vi "DGHD5331_timestamp.vi"() -> ()   [LabVIEW 2014]
uses:
  <vilib>/Instr/_visa.llb/VISA Configure Serial Port (Instr).vi
  <vilib>/Utility/file.llb/Write To Spreadsheet File (string).vi
  <vilib>/Utility/file.llb/Write To Spreadsheet File (DBL).vi
panel:
  out "Time/Date":string
  out "Waveform Chart":dynamicdata(graph)
  out "Data Read":string
  out "Exp time (sec)":dbl
  out "Bytes Read":u32
  in  "Comm Port":refnum<visa-resource-name>
  in  "Loop Timer":u32=500 min=500 max=5000 step=500
  in  "stop":bool
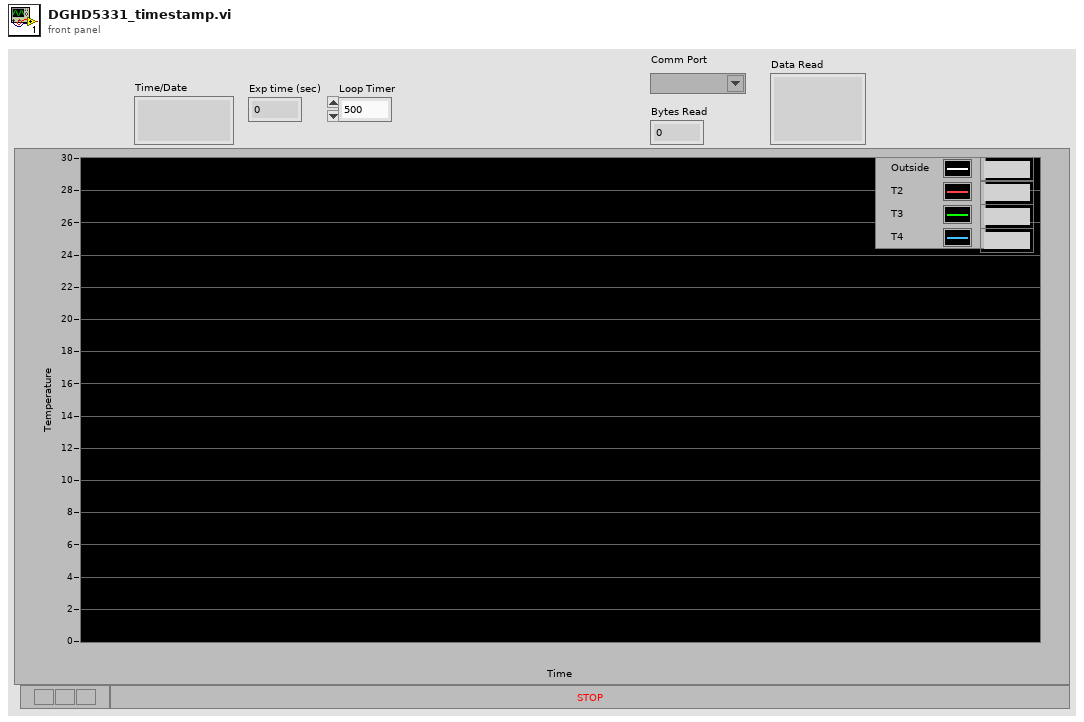
[diagram p1: front panel]
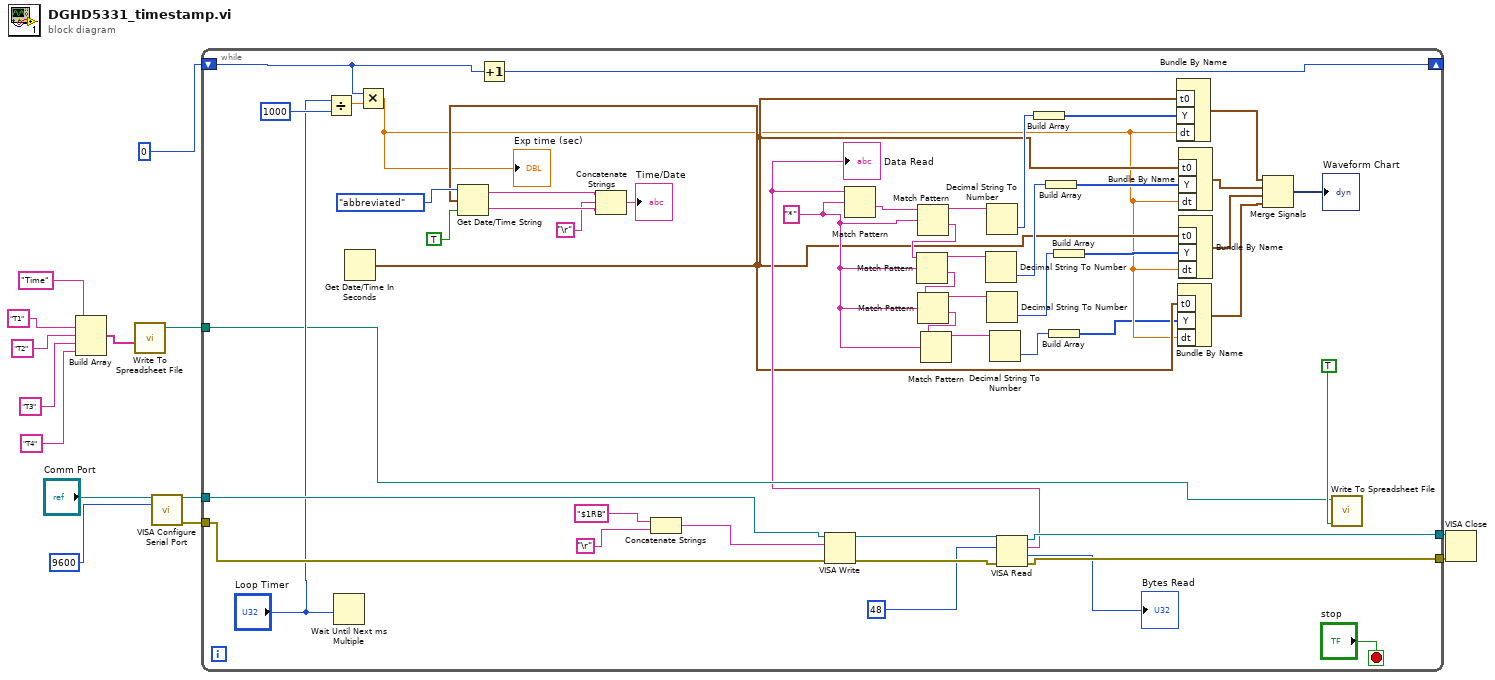
[diagram p0: block diagram]
diagram:
  n1 = Build Array("Time", "T1", "T2", "T3", "T4") -> (w3:string[])
  n2 = call-poly <vilib>:"Write To Spreadsheet File.vi"("1D data"=w3) -> ("new file path (Not A Path if cancelled)"=w1:path)  [unwired: 7 in]
  n3 = call-poly "VISA Configure Serial Port"("VISA resource name"="Comm Port", "baud rate (9600)"=9600) -> ("VISA resource name out"=w13:refnum<visa-resource-name>, "error out"=w11:errorcluster)  [unwired: 12 in]
  n4 = while {
    tunnel: w13 -> [w63]
    tunnel: w11 -> [w62]
    tunnel: [w59] -> w10
    tunnel: [w58] -> w9
    shift-right: [w39] -> _
    shift-left: 0 -> [w50]
    tunnel: w1 -> [w38]
    stop <- "stop" stop-if-true
    w43 = "*"
    n5 = Divide(x="Loop Timer", y=1000) -> (x/y=w52:dbl)
    n6 = Wait Until Next ms Multiple(millisecond multiple="Loop Timer") -> ()  [unwired: 1 out]
    n7 = Get Date/Time In Seconds() -> (seconds since 1Jan1904=w27:timestamp)
    n8 = Multiply(x=w50, y=w52) -> (x*y=w26:dbl)
    "Exp time (sec)" <- w26
    n9 = Get Date/Time String(date format (0)=enum16{"short", "long", "abbreviated"}."abbreviated", seconds (now)=w27, want seconds? (F)=TRUE) -> (date string=w18:string, time string=w17:string)
    n10 = Increment(x=w50) -> (x+1=w39:i32)
    n11 = Concatenate Strings(w18, "\r", w17) -> (→"Time/Date":string)
    n12 = Concatenate Strings("$1RB", "\r") -> (w54:string)
    n13 = VISA Write(VISA resource name=w63, write buffer=w54, error in (no error)=w62) -> (VISA resource name out=w61:refnum<visa-resource-name>, error out=w60:errorcluster)  [unwired: 1 out]
    n14 = VISA Read(VISA resource name=w61, byte count=u32 48 ("Bytes Read"), error in (no error)=w60) -> (VISA resource name out=w59:refnum<visa-resource-name>, read buffer=w37:string, return count=→"Bytes Read":u32, error out=w58:errorcluster)
    "Data Read" <- w37
    n15 = Match Pattern(string=w37, regular expression=w43) -> (after substring=w49:string)  [unwired: 1 in, 3 out]
    n16 = Match Pattern(string=w49, regular expression=w43) -> (before substring=w48:string, after substring=w46:string)  [unwired: 1 in, 2 out]
    n17 = Match Pattern(string=w46, regular expression=w43) -> (before substring=w47:string, after substring=w42:string)  [unwired: 1 in, 2 out]
    n18 = Match Pattern(string=w42, regular expression=w43) -> (before substring=w45:string, after substring=w41:string)  [unwired: 1 in, 2 out]
    n19 = Match Pattern(string=w41, regular expression=w43) -> (before substring=w44:string)  [unwired: 1 in, 3 out]
    n20 = Decimal String To Number(string=w47) -> (number=w32:i32)  [unwired: 2 in, 1 out]
    n21 = Decimal String To Number(string=w48) -> (number=w33:i32)  [unwired: 2 in, 1 out]
    n22 = Decimal String To Number(string=w45) -> (number=w29:i32)  [unwired: 2 in, 1 out]
    n23 = Decimal String To Number(string=w44) -> (number=w25:i32)  [unwired: 2 in, 1 out]
    n24 = Build Array(w33) -> (w31:i32[])
    n25 = Build Array(w32) -> (w30:i32[])
    n26 = Build Array(w25) -> (w24:i32[])
    n27 = Build Array(w29) -> (w28:i32[])
    n28 = Bundle By Name("t0"=w27, "Y"=w31, "dt"=w26) -> (w23:waveform(i32))  [unwired: 1 in]
    n29 = Bundle By Name("t0"=w27, "Y"=w24, "dt"=w26) -> (w20:waveform(i32))  [unwired: 1 in]
    n30 = Bundle By Name("t0"=w27, "Y"=w30, "dt"=w26) -> (w22:waveform(i32))  [unwired: 1 in]
    n31 = Bundle By Name("t0"=w27, "Y"=w28, "dt"=w26) -> (w21:waveform(i32))  [unwired: 1 in]
    n32 = Merge Signals(w23, w22, w21, w20) -> (→"Waveform Chart":dynamicdata)
    n33 = call-poly <vilib>:"Write To Spreadsheet File.vi"("append to file? (new file:F)"=TRUE, "file path (dialog if empty)"=w38) -> ()  [unwired: 6 in, 1 out]
  }
  n34 = VISA Close(VISA resource name=w10, error in (no error)=w9) -> ()  [unwired: 1 out]
